vi "testKeithleyScript.vi"() -> ()   [LabVIEW 2009, in "run.lvlib"]
uses:
  run.lvlib
  Channels/VoltOutput/K2602/K2602.lvclass
  Channels/VoltOutput/AnalogOutput.lvclass
panel:
  out "script":string
  in  "physical channels":string="K2602a_Ao_00"
  in  "stop":bool
  in  "data":dbl[][][](array[numeric])=[[[0.56, 1.0], [2.0, 3.0]]]
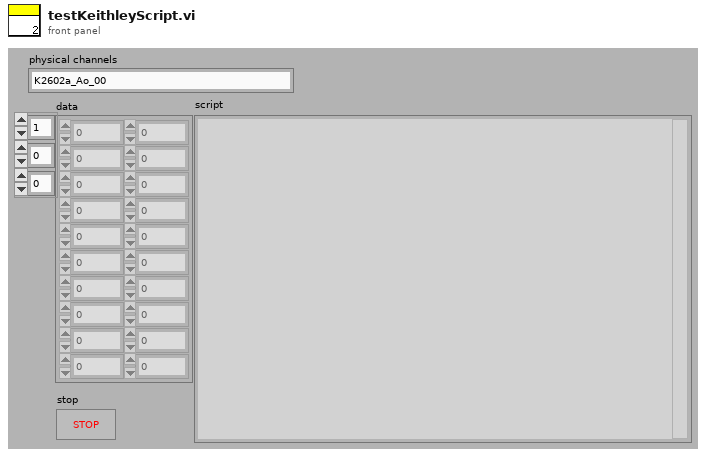
[diagram p1: front panel]
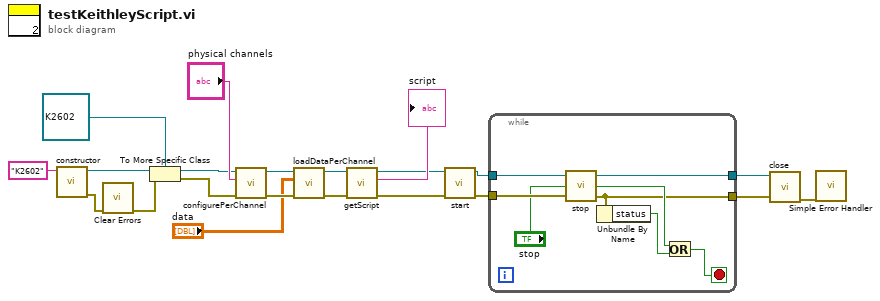
[diagram p0: block diagram]
diagram:
  n1 = call "constructor.vi"("deviceName"="K2602") -> ("error out"=w2:errorcluster, "AnalogOutput out"=w7:refnum<class "AnalogOutput.lvclass">)  [unwired: 9 in]
  n2 = call <vilib>:"Clear Errors.vi"("error in (no error)"=w2) -> ("error out"=w1:errorcluster)  [unwired: 6 in]
  n3 = To More Specific Class(target class=refnum<class "K2602.lvclass"> refnum ("Hardware:Channels.lvlib:K2602.lvclass"), reference=w7, error in=w1) -> (specific class reference=w5:refnum<class "K2602.lvclass">, error out=w4:errorcluster)
  n4 = call-dynamic "configurePerChannel.vi"("error in (no error)"=w4, "physical channels"="physical channels", "K2602 in"=w5) -> ("error out"=w19:errorcluster, "K2602 out"=w20:refnum<class "K2602.lvclass">)  [unwired: 7 in]
  n5 = call-dynamic "loadDataPerChannel.vi"("error in (no error)"=w19, "data"="data", "K2602 in"=w20) -> ("error out"=w16:errorcluster, "K2602 out"=w17:refnum<class "K2602.lvclass">)  [unwired: 7 in]
  n6 = call "getScript.vi"("error in (no error)"=w16, "K2602 in"=w17) -> ("error out"=w13:errorcluster, "script"=→"script":string, "K2602 out"=w14:refnum<class "K2602.lvclass">)  [unwired: 7 in]
  n7 = call-dynamic "start.vi"("error in (no error)"=w13, "K2602 in"=w14) -> ("error out"=w11:errorcluster, "K2602 out"=w12:refnum<class "K2602.lvclass">)  [unwired: 8 in]
  n8 = while {
    tunnel: w12 -> [w29]
    tunnel: w11 -> [w28]
    tunnel: [w23] -> w10
    tunnel: [w22] -> w9
    stop <- w26 stop-if-true
    n9 = call-dynamic "stop.vi"("error in (no error)"=w28, "stop"="stop", "K2602 in"=w29) -> ("error out"=w22:errorcluster, "Stopped"=w25:bool, "K2602 out"=w23:refnum<class "K2602.lvclass">)
    n10 = Unbundle By Name(w22) -> ("status"=w24:bool)
    n11 = Or(x=w25, y=w24) -> (x .or. y?=w26:bool)
  }
  n12 = call-dynamic "close.vi"("error in (no error)"=w9, "K2602 in"=w10) -> ("error out"=w8:errorcluster)  [unwired: 9 in]
  n13 = call <vilib>:"Simple Error Handler.vi"("error in (no error)"=w8) -> ()  [unwired: 4 in, 5 out]
